vi "Pfeiffer-RVC300.close valve.vi"(0 "i ref in":refnum<vi>, 3 "ms timeout (10000)":i32=10000, 5 "error in (no error)":errorcluster) -> (14 "i ref out":refnum<vi>, 17 "timed out":bool, 19 "error out":errorcluster)   [LabVIEW 2014, in "Pfeiffer-RVC300.lvlib"]
doc: "Closes the valve.\n\nLicense Agreement for this software:\n\nCopyright (C)\nMax-Planck-Institut für Kernphysik\nSaupfercheckweg 1\n69117 Heidelberg\nGermany\n\nContact: christopher.borgmann@mpi-hd.mpg.de\n\nThis program is free software: you can redistribute it and/or modify \nit under the terms of the GNU General Public License as published by\nthe Free Software Foundation, either version 3 of the License, or\n(at your option) any later version.\n\nThis program is distributed in the hope that it will be useful,\nbut WITHOUT ANY WARRANTY; without even the implied warranty of\nMERCHANTABILITY or FITNESS FOR A PARTICULAR PURPOSE. See the\nGNU General Public License for more details.\n\nYou should have received a copy of the GNU General Public License\nalong with this program. If not, see <http://www.gnu.org/licenses/>.\n\nMax-Planck-Institut für Kernphysik\nSaupfercheckweg 1, 69117 Heidelberg, Germany\nFor all questions and ideas contact: christopher.borgmann@mpi-hd.mpg.de\nLast update: 08.07.2010"
uses:
  Pfeiffer-RVC300.lvlib
  CSCore/CSApplicationBaseClasses/DeviceBase/DeviceBase.lvlib
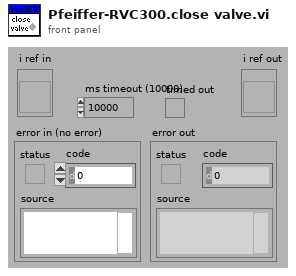
[diagram p1: front panel]
types:
  T1 = typedef "Pfeiffer-RVC300.lvlib/Pfeiffer-RVC300.i attribute.ctl" = cluster{"interfaceInitialized":bool, "VISAResource":refnum<visa-resource-name>, "WaitingTime":u32, "nomValues":T2, "actValues":T2}
  T2 = typedef "Pfeiffer-RVC300.lvlib/Pfeiffer-RVC300.parameters.ctl" = cluster{"regulationMode":T3, "valveType":string, "sensorType":string, "valveState":string, "flow":dbl, "pressure":dbl, "serviceIDs":cluster{"regulationModeID":i32, "valveTypeID":i32, "sensorTypeID":i32, "valveStateID":i32, "flowID":i32, "pressureID":i32}}
  T3 = typedef "Pfeiffer-RVC300.lvlib/Pfeiffer-RVC300.regulation mode.ctl" = enum16{"unknown", "Pressure", "Flow", "Wait"}
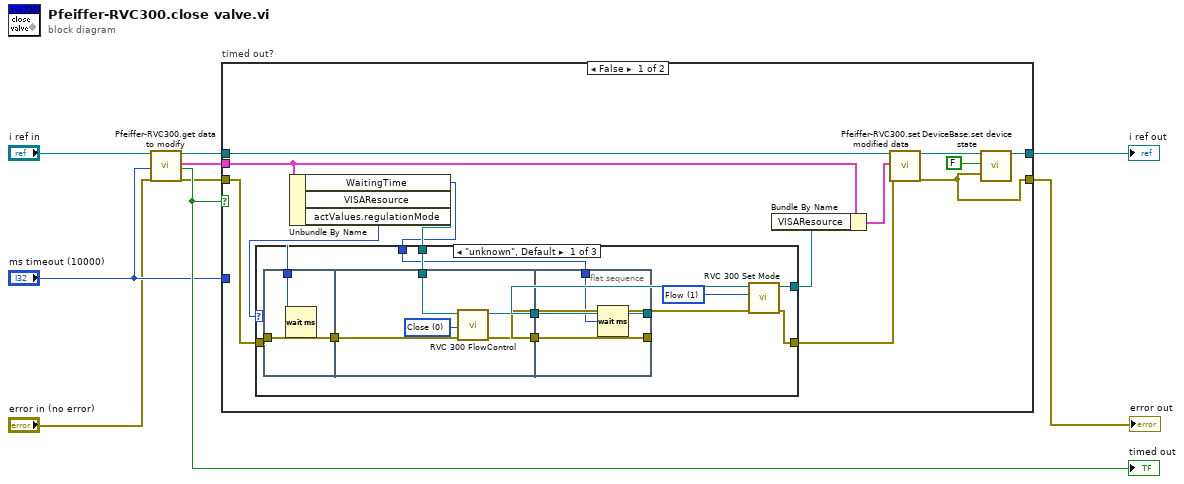
[diagram p0: block diagram]
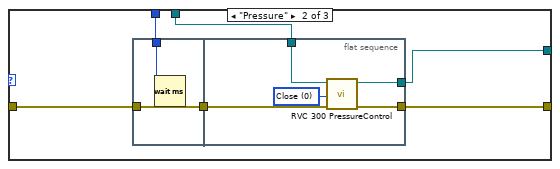
[diagram p2: hidden frame]
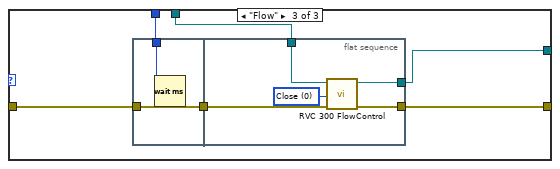
[diagram p3: hidden frame]
diagram:
  n1 = call "Pfeiffer-RVC300.get data to modify.vi"("i ref in"="i ref in", "ms timeout (10000)"="ms timeout (10000)", "error in (no error)"="error in (no error)") -> ("i ref out"=w3:refnum<vi>, "i attribute"=w1:T1, "timed out"=w6:bool, "error out"=w2:errorcluster)  [unwired: 13 in]
  "timed out" <- w6
  n2 = case "timed out?" shown="False" w6 {
    tunnel: [w19 w71] -> w8
    tunnel: w3 -> [w22 w71]
    tunnel: [w17 w70] -> w7
    tunnel: w2 -> [w16 w70]
    tunnel: w1 -> [w13 _]
    tunnel: "ms timeout (10000)" -> [_ _]
    frame False {
      n3 = Unbundle By Name(w13) -> ("WaitingTime"=w11:u32, "VISAResource"=w12:refnum<visa-resource-name>, "actValues.regulationMode"=w10:T3)
      n4 = case shown="\"unknown\", Default" w10 {
        tunnel: w16 -> [w30 w48 w61]
        tunnel: [w29 w47 w60] -> w15
        tunnel: [w26 w46 w59] -> w14
        tunnel: w12 -> [w24 w45 w58]
        tunnel: w11 -> [w23 w44 w57]
        frame "unknown", Default {
          w25 = u16 1 items=["Pressure", "Flow", "Wait"] ("Mode")
          n5 = flat-sequence {
            tunnel: w30 -> [w35]
            tunnel: [w35] -> w33
            tunnel: w23 -> [w34]
            tunnel: [w39] -> w32
            tunnel: [w37] -> w31
            tunnel: w33 -> [w40]
            tunnel: w24 -> [w36]
            tunnel: [w42] -> w27
            tunnel: [w43] -> w28
            tunnel: w32 -> [w43]
            tunnel: w31 -> [w42]
            tunnel: w23 -> [w41]
            frame #0 {
              n6 = Wait (ms)(milliseconds to wait=w34) -> ()  [unwired: 1 out]
            }
            frame #1 {
              w38 = u16 0 items=["Close", "Open", "Control"] ("Action")
              n7 = call "RVC 300 FlowControl.vi"("error in"=w40, "Action"=w38, "Resource Name"=w36) -> ("error out"=w37:errorcluster, "Resource Name out"=w39:refnum<visa-resource-name>)  [unwired: 6 in, 1 out]
            }
            frame #2 {
              n8 = Wait (ms)(milliseconds to wait=w41) -> ()  [unwired: 1 out]
            }
          }
          n9 = call "RVC 300 Set Mode.vi"("error in"=w27, "Mode"=w25, "Resource Name"=w28) -> ("error out"=w29:errorcluster, "Resource Name out"=w26:refnum<visa-resource-name>)  [unwired: 3 in]
        }
        frame "Pressure" {
          n10 = flat-sequence {
            tunnel: w48 -> [w51]
            tunnel: [w51] -> w49
            tunnel: w44 -> [w50]
            tunnel: w49 -> [w56]
            tunnel: w45 -> [w54]
            tunnel: [w53] -> w47
            tunnel: [w52] -> w46
            frame #0 {
              n11 = Wait (ms)(milliseconds to wait=w50) -> ()  [unwired: 1 out]
            }
            frame #1 {
              w55 = u16 0 items=["Close", "Open", "Control"] ("Action")
              n12 = call "RVC 300 PressureControl.vi"("error in"=w56, "Action"=w55, "Resource Name"=w54) -> ("error out"=w53:errorcluster, "Resource Name out"=w52:refnum<visa-resource-name>)  [unwired: 3 in]
            }
          }
        }
        frame "Flow" {
          n13 = flat-sequence {
            tunnel: w61 -> [w64]
            tunnel: [w64] -> w62
            tunnel: w57 -> [w63]
            tunnel: w62 -> [w69]
            tunnel: w58 -> [w67]
            tunnel: [w66] -> w60
            tunnel: [w65] -> w59
            frame #0 {
              n14 = Wait (ms)(milliseconds to wait=w63) -> ()  [unwired: 1 out]
            }
            frame #1 {
              w68 = u16 0 items=["Close", "Open", "Control"] ("Action")
              n15 = call "RVC 300 FlowControl.vi"("error in"=w69, "Action"=w68, "Resource Name"=w67) -> ("error out"=w66:errorcluster, "Resource Name out"=w65:refnum<visa-resource-name>)  [unwired: 6 in, 1 out]
            }
          }
        }
      }
      n16 = Bundle By Name(cluster=w13, "VISAResource"=w14) -> (w21:T1)
      n17 = call "Pfeiffer-RVC300.set modified data.vi"("i ref in"=w22, "i attribute"=w21, "error in (no error)"=w15) -> ("i ref out"=w20:refnum<vi>, "error out"=w17:errorcluster)  [unwired: 15 in]
      n18 = call "DeviceBase.set device state.vi"("i ref in"=w20, "implicit"=FALSE, "device error"=w17) -> ("i ref out"=w19:refnum<vi>)  [unwired: 14 in, 2 out]
    }
    frame True {
    }
  }
  "error out" <- w7
  "i ref out" <- w8
